vi "Macro Initialize.vi"(7 "Front Panel Window:Open":bool, 8 "error in (no error)":errorcluster, 11 "UI ActorTop in":refnum<class "UIActorTop.lvclass">) -> (0 "error out":errorcluster, 3 "UI ActorTop out":refnum<class "UIActorTop.lvclass">)   [LabVIEW 2021, in "AbstractActorTemplate.lvlib" / "UIActorTop.lvclass"]
doc: "Macro: Initialize\nevery children class override this vi and rewrite it. put itseft Messages in this vi.\n2015-03-18 16:07:01\n蒋松\njiangsong@outlook.com"
uses:
  <userlib>/John_Lib/AbstractActorTemplate/AbstractActorTemplate/UIActorTop.lvclass
  <userlib>/John_Lib/AbstractActorTemplate/AbstractActorTemplate/UIActorTop.lvclass/UIActorTop.ctl
  <userlib>/sushu/sushu.lvlib
  C:/Program Files (x86)/National Instruments/LabVIEW 2021/vi.lib/ActorFramework/Actor/Actor.lvclass
  C:/Program Files (x86)/National Instruments/LabVIEW 2021/user.lib/John_Lib/AbstractActorTemplate/AbstractActorTemplate/UIActorTop.lvclass
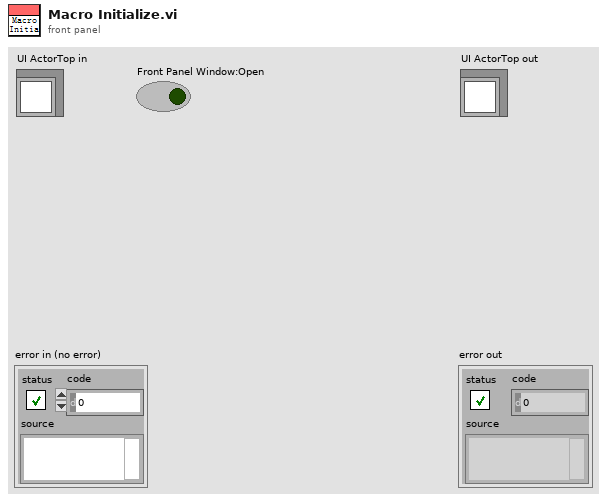
[diagram p1: front panel]
types:
  T1 = enum32{"invalid app kind", "Development System", "Run Time System", "Student Edition", "Embedded LabVIEW", "Evaluation", "Custom"}
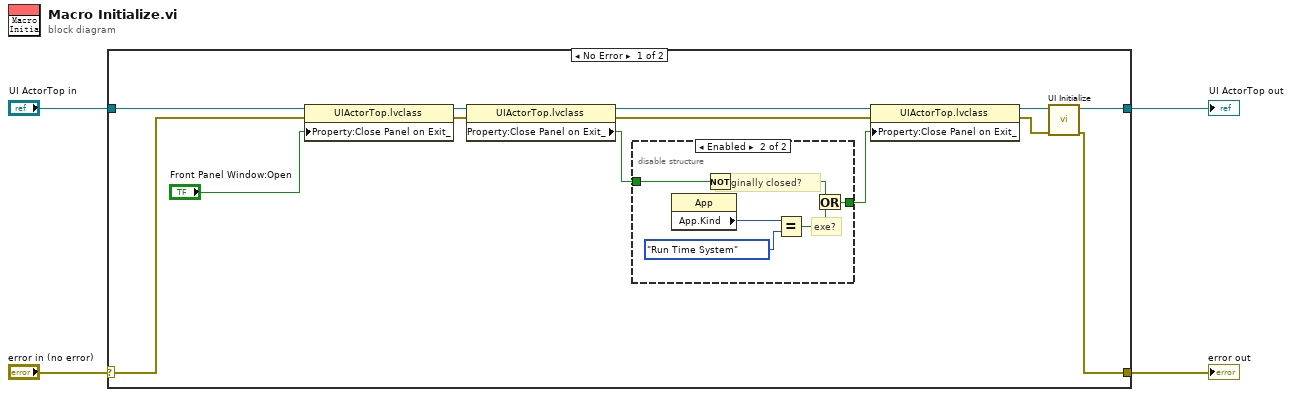
[diagram p0: block diagram]
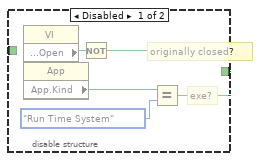
[diagram p2: hidden frame]
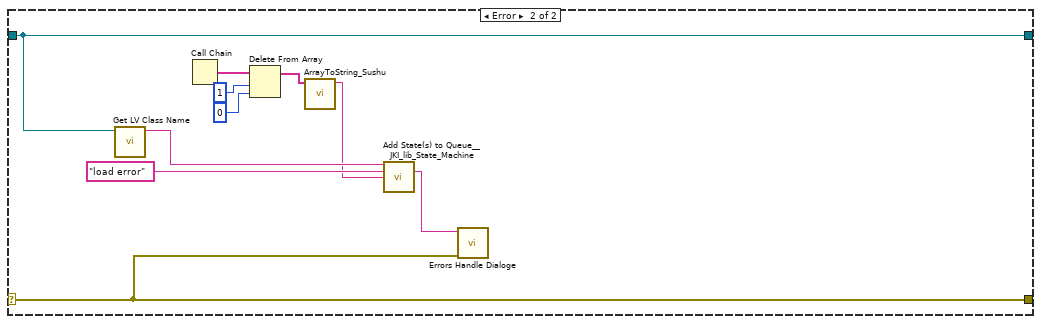
[diagram p3: hidden frame]
diagram:
  n1 = case shown="No Error" "error in (no error)" {
    selector: "error in (no error)" -> [w10 w32]
    tunnel: [w5 w32] -> w3
    tunnel: [w7 w33] -> w1
    tunnel: "UI ActorTop in" -> [w9 w33]
    frame No Error {
      n2 = property class="UIActorTop.lvclass"(reference=w9, error in=w10, "Property:Close Panel on Exit_"="Front Panel Window:Open") -> (reference out=w12:refnum<class "UIActorTop.lvclass">, error out=w11:errorcluster)
      n3 = property class="UIActorTop.lvclass"(reference=w12, error in=w11) -> (reference out=w15:refnum<class "UIActorTop.lvclass">, error out=w13:errorcluster, "Property:Close Panel on Exit_"=w16:bool)
      n4 = disable-structure shown="Enabled" {
        disable-tunnel: [w18 w25] -> w14
        disable-tunnel: w16 -> [_ w24]
        frame Disabled {
          # "originally closed?"
          # "exe?"
          n5 = property class="VI"() -> ("Front Panel.Open"=w19:bool)  [unwired: 2 in, 2 out]
          n6 = property class="App"() -> ("App.Kind"=w20:T1)  [unwired: 2 in, 2 out]
          n7 = Not(x=w19) -> (.not. x?=w22:bool)
          n8 = Equal?(x=w20, y=T1."Run Time System" ("Application:Kind")) -> (x = y?=w23:bool)
          n9 = Or(x=w22, y=w23) -> (x .or. y?=w18:bool)
        }
        frame Enabled {
          # "originally closed?"
          # "exe?"
          n10 = property class="App"() -> ("App.Kind"=w26:T1)  [unwired: 2 in, 2 out]
          n11 = Not(x=w24) -> (.not. x?=w28:bool)
          n12 = Equal?(x=w26, y=T1."Run Time System" ("Application:Kind")) -> (x = y?=w29:bool)
          n13 = Or(x=w28, y=w29) -> (x .or. y?=w25:bool)
        }
      }
      n14 = property class="UIActorTop.lvclass"(reference=w15, error in=w13, "Property:Close Panel on Exit_"=w14) -> (reference out=w8:refnum<class "UIActorTop.lvclass">, error out=w6:errorcluster)
      n15 = call-dynamic "UI Initialize.vi"("error in (no error)"=w6, "UI ActorTop in"=w8) -> ("error out"=w5:errorcluster, "UI ActorTop out"=w7:refnum<class "UIActorTop.lvclass">)  [unwired: 8 in]
    }
    frame Error {
      n16 = call <vilib>:"Get LV Class Name.vi"("object"=w33) -> ("class name"=w38:string)  [unwired: 9 in, 1 out]
      n17 = Call Chain() -> (call chain=w31:string[])
      n18 = Delete From Array(array=w31, length=1, index=0) -> (array with subset deleted=w30:string[])  [unwired: 1 out]
      n19 = call <userlib>:"ArrayToString_Sushu.vi"("Array"=w30) -> ("String"=w34:string)  [unwired: 10 in]
      n20 = call <vilib>:"Add State(s) to Queue__JKI_lib_State_Machine.vi"("State(s) in Front (\"\")"=w38, "State(s) in (\"\")"="load error" ("State(s) in (\"\")"), "State(s) at Back (\"\")"=w34) -> ("States Out"=w39:string)  [unwired: 12 in]
      n21 = call <userlib>:"Errors Handle Dialoge.vi"("error in (no error)"=w32, "Message"=w39) -> ()  [unwired: 8 in, 2 out]
    }
  }
  "error out" <- w3
  "UI ActorTop out" <- w1
